vi "Start Block Status.vi"(4 "Started":bool, 6 "Init":bool, 8 "Block State":T2, 10 "i":i32, 11 "Status Queue In":refnum<queue>) -> (1 "Status":T1={"State"=enum."Init", "i"=0, "Init"=FALSE, "Started"=FALSE, "Action"=enum."N/A"}, 3 "Status Queue":refnum<queue>)   [LabVIEW 2020, in "FlexBlocks.lvlib"]
uses:
  FlexBlocks.lvlib
  Block State.ctl
  Block Status.ctl
  Run Action.ctl
  Block Status with Error.ctl
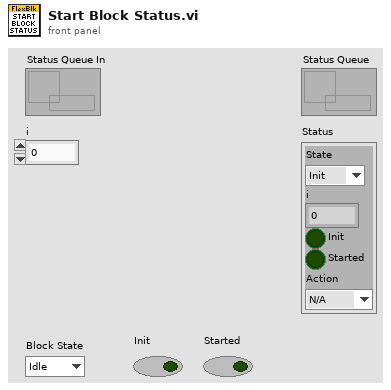
[diagram p1: front panel]
types:
  T1 = typedef "FlexBlocks.lvlib/Block Status.ctl" = cluster{"State":T2, "i":i32, "Init":bool, "Started":bool, "Action":T3}
  T2 = typedef "FlexBlocks.lvlib/Block State.ctl" = enum16{"Idle", "Init", "Start", "Run", "Stop"}
  T3 = typedef "FlexBlocks.lvlib/Run Action.ctl" = enum16{"N/A", "Read", "Work", "Write"}
  T4 = typedef "FlexBlocks.lvlib/Block Status with Error.ctl" = cluster{"Status":T1, "Error":errorcluster}
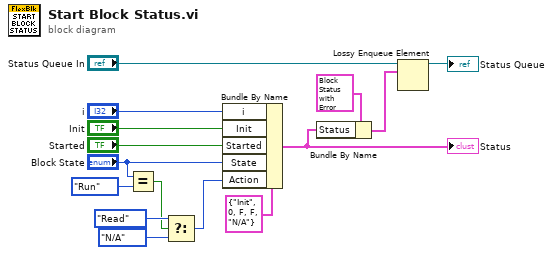
[diagram p0: block diagram]
diagram:
  n1 = Equal?(x="Block State", y=Block_State."Run") -> (x = y?=w7:bool)
  n2 = Select(t=Run_Action."Read" ("Work Action"), s=w7, f=Run_Action."N/A" ("Work Action")) -> (s? t:f=w6:T3)
  n3 = Bundle By Name(cluster=T1 {"State"=enum."Init", "i"=0, "Init"=FALSE, "Started"=FALSE, "Action"=enum."N/A"} ("Status"), "i"="i", "Init"="Init", "Started"="Started", "State"="Block State", "Action"=w6) -> (w2:T1)
  "Status" <- w2
  n4 = Bundle By Name(cluster=T4 {"Status"={"State"=enum."Init", "i"=0, "Init"=FALSE, "Started"=FALSE, "Action"=enum."N/A"}, "Error"={"status"=FALSE, "code"=0, "source"=""}} ("Block Status with Error"), "Status"=w2) -> (w1:T4)
  n5 = Lossy Enqueue Element(queue="Status Queue In", element=w1) -> (queue out=→"Status Queue":refnum<queue>)  [unwired: 1 in, 3 out]
